vi "PSU Status (Read).vi"(6 "ISOBUS address":T3=-1 caption="ISOBUS address (-1)", 8 "error in":errorcluster, 11 "Mercury Reference In":T4) -> (0 "error out":errorcluster, 1 "Status Hex value":i32, 2 "PSU Act Stat":T1 caption="PSU Status", 3 "Mercury Reference Out":T4, 4 "Valid?":T2, 5 "Status":string)   [LabVIEW 2013, in "Mercury iXX.lvlib" / "Magnet.lvlib"]
doc: "Acquire the most recent PSU action status signal."
uses:
  Magnet.lvlib
  Mercury iXX.lvlib
  Private/Controls/Command Verbs.ctl
  Controls/Is Valid LED.ctl
  Controls/Comms Transport Layer.ctl
  Controls/Mercury Reference.ctl
  Controls/ISOBus Address.ctl
  Private/Controls/Query Dynamic Reference.ctl
  Controls/PSU Actions.ctl
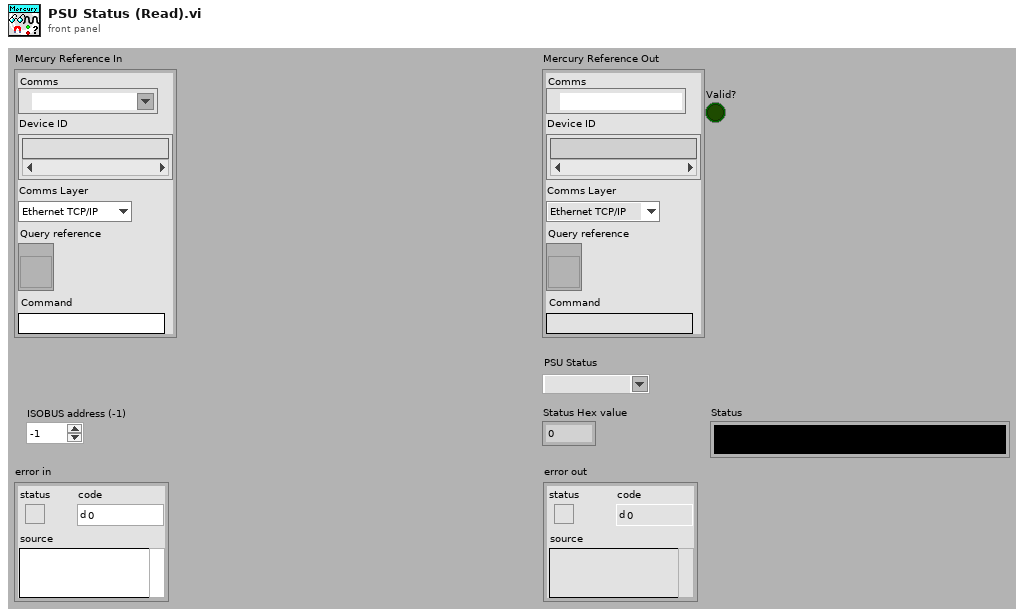
[diagram p1: front panel]
types:
  T1 = typedef "Mercury iXX.lvlib/Magnet.lvlib/PSU Actions.ctl" = string
  T2 = typedef "Mercury iXX.lvlib/Is Valid LED.ctl" = bool
  T3 = typedef "Mercury iXX.lvlib/ISOBus Address.ctl" = i32
  T4 = typedef "Mercury iXX.lvlib/Mercury Reference.ctl" = cluster{"Comms":refnum<visa-resource-name>, "Device ID":string[], "Comms Layer":T5, "Command":string, "Query reference":T6}
  T5 = typedef "Mercury iXX.lvlib/Comms Transport Layer.ctl" = enum16{"Ethernet TCP/IP", "USB", "ISOBus - RS-232", "GPIB"}
  T6 = typedef "Mercury iXX.lvlib/Query Dynamic Reference.ctl" = refnum<vi>
  T7 = typedef "Mercury iXX.lvlib/Command Verbs.ctl" = string
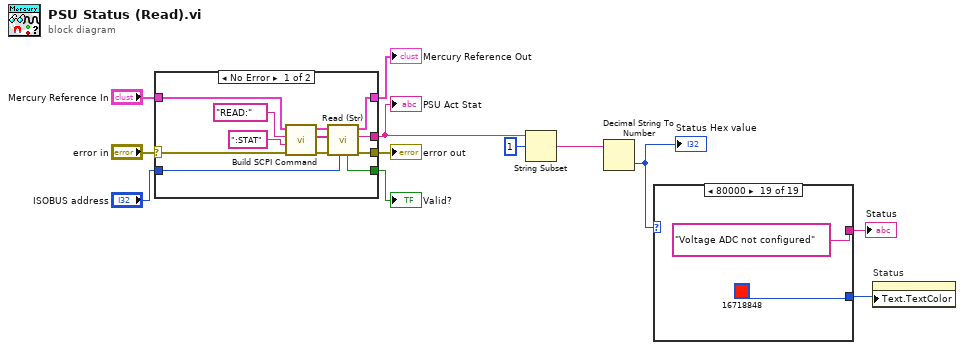
[diagram p0: block diagram]
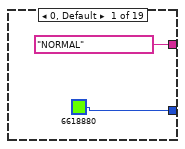
[diagram p2: hidden frame]
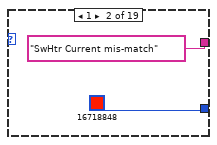
[diagram p3: hidden frame]
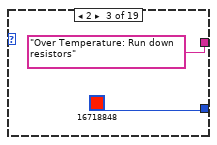
[diagram p4: hidden frame]
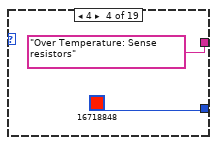
[diagram p5: hidden frame]
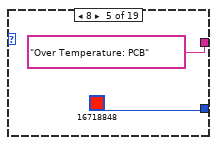
[diagram p6: hidden frame]
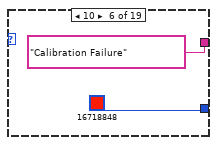
[diagram p7: hidden frame]
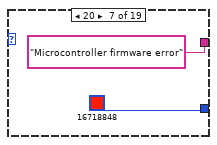
[diagram p8: hidden frame]
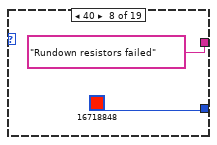
[diagram p9: hidden frame]
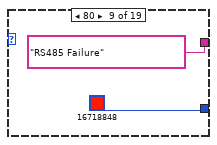
[diagram p10: hidden frame]
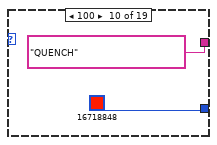
[diagram p11: hidden frame]
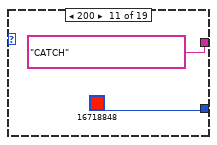
[diagram p12: hidden frame]
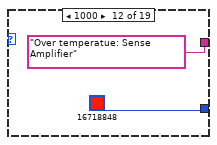
[diagram p13: hidden frame]
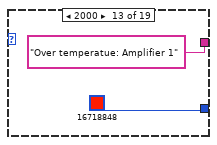
[diagram p14: hidden frame]
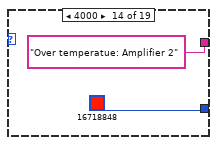
[diagram p15: hidden frame]
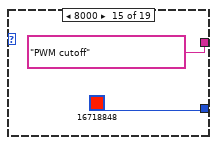
[diagram p16: hidden frame]
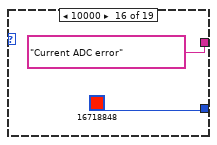
[diagram p17: hidden frame]
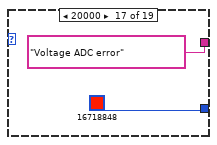
[diagram p18: hidden frame]
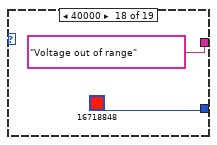
[diagram p19: hidden frame]
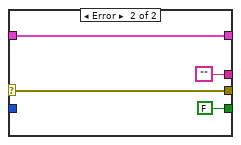
[diagram p20: hidden frame]
diagram:
  n1 = case shown="No Error" "error in" {
    selector: "error in" -> [w13 w27]
    tunnel: [w24 w28] -> w12
    tunnel: [w23 w27] -> w11
    tunnel: [w22 T2 FALSE ("Valid?")] -> w10
    tunnel: "ISOBUS address" -> [w21 _]
    tunnel: [w20 ""] -> w3
    tunnel: "Mercury Reference In" -> [w17 w28]
    frame No Error {
      n2 = call "Build SCPI Command.vi"("error in"=w13, "Noun(s)"=":STAT" ("Command"), "Verb"=T7 "READ:", "Mercury Reference In"=w17) -> ("error out"=w15:errorcluster, "SCPI Message(s)"=w14:string[], "Mercury Reference Out"=w16:T4)  [unwired: 5 out]
      n3 = call "Read (Str).vi"("ISOBUS address"=w21, "error in"=w15, "SCPI Message(s)"=w14, "Mercury Reference In"=w16) -> ("error out"=w23:errorcluster, "Response"=w20:string, "Mercury Reference Out"=w24:T4, "Valid?"=w22:T2)  [unwired: 4 out]
    }
    frame Error {
    }
  }
  "Mercury Reference Out" <- w12
  "error out" <- w11
  "Valid?" <- w10
  "PSU Act Stat" <- w3
  n4 = String Subset(string=w3, offset (0)=1) -> (substring=w1:string)  [unwired: 1 in]
  n5 = Decimal String To Number(string=w1) -> (number=w6:i32)  [unwired: 2 in, 1 out]
  "Status Hex value" <- w6
  n6 = case shown="80000" w6 {
    tunnel: ["NORMAL" "SwHtr Current mis-match" "Over Temperature: Run down resistors" "Over Temperature: Sense resistors" "Over Temperature: PCB" "Calibration Failure" "Microcontroller firmware error" "Rundown resistors failed" "RS485 Failure" "QUENCH" "CATCH" "Over temperatue: Sense Amplifier" "Over temperatue: Amplifier 1" "Over temperatue: Amplifier 2" "PWM cutoff" "Current ADC error" "Voltage ADC error" "Voltage out of range" "Voltage ADC not configured"] -> w5
    tunnel: [u32 6618880 u32 16718848 u32 16718848 u32 16718848 u32 16718848 u32 16718848 u32 16718848 u32 16718848 u32 16718848 u32 16718848 u32 16718848 u32 16718848 u32 16718848 u32 16718848 u32 16718848 u32 16718848 u32 16718848 u32 16718848 u32 16718848] -> w4
    frame 0, Default {
    }
    frame 1 {
    }
    frame 2 {
    }
    frame 4 {
    }
    frame 8 {
    }
    frame 10 {
    }
    frame 20 {
    }
    frame 40 {
    }
    frame 80 {
    }
    frame 100 {
    }
    frame 200 {
    }
    frame 1000 {
    }
    frame 2000 {
    }
    frame 4000 {
    }
    frame 8000 {
    }
    frame 10000 {
    }
    frame 20000 {
    }
    frame 40000 {
    }
    frame 80000 {
    }
  }
  "Status" <- w5
  n7 = property on="Status" class="Str"("Text.TextColor"=w4) -> ()  [unwired: 2 in, 2 out]
